vi "Path Variant to Path Array.vi"(8 "error in":errorcluster, 10 "Paths":variant) -> (0 "error out":errorcluster, 2 "Paths":string[](array[string]))   [LabVIEW 2019, in "LV-Data.PGSQL.lvclass"]
uses:
  LV-Data.PGSQL.lvclass
  Typedefs/Errors--enum.ctl
  <vilib>/Utility/Data Type/NI_Data Type.lvlib
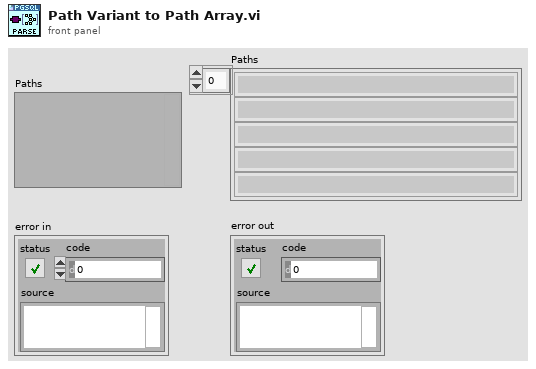
[diagram p1: front panel]
types:
  T1 = typedef "NI_Data Type.lvlib/Data Type.ctl" = enum8{"Invalid Type", "Void", "I8", "I16", "I32", "I64", "U8", "U16", "U32", "U64", "Single Float", "Double Float", "Extended Float", "Single Complex", "Double Complex", "Extended Complex", "Enum U8", "Enum U16", "Enum U32", "Enum U64", "Single Float With Unit", "Double Float With Unit", "Extended Float With Unit", "Single Complex with Unit", "Double Complex with Unit", "Extended Complex with Unit", "Boolean", "String", "Path", "Picture", "Tag", "Array", "Cluster", "Variant", "LV Variant", "Waveform", "Timestamp", "Digital Waveform", "Digital Data", "ExpressData", "Refnum", "External Data", "VI", "Poly VI", "LabVIEW Class Instance", "Fixed Point", "Set Collection", "Map Collection"}
  T2 = typedef "LV-Data.PGSQL.lvclass/Errors--enum.ctl" = enum16{"0: None", "5005: Path Type Not Supported", "5006: Number of Variables", "5007: Number of data points", "5008: Cannot write two data points", "5030: Start and End Times Identical", "5031: Input is not wholly", "5032: Undefined Timestamps", "5033: Bad path or paths", "5040: Invalid Instrument Name", "5050: Column can only hold string", "5051: Column can only hold bool", "5052: Column can only hold double", "5053: Column can only hold int"}
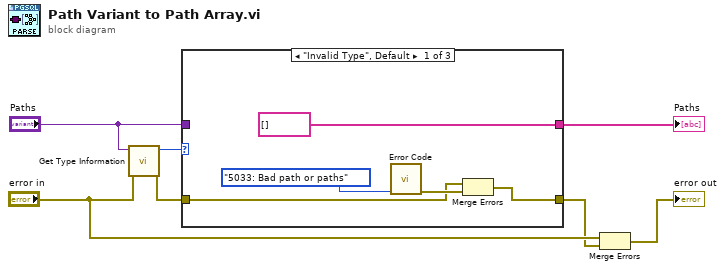
[diagram p0: block diagram]
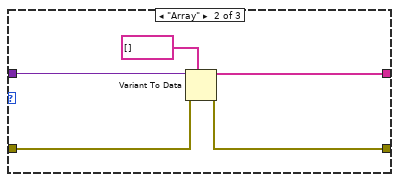
[diagram p2: hidden frame]
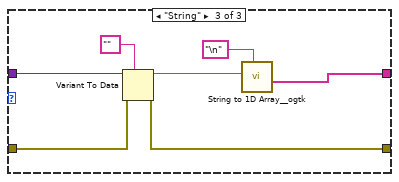
[diagram p3: hidden frame]
diagram:
  n1 = call <vilib>:"Get Type Information.vi"("error in (no error)"="error in", "variant"="Paths") -> ("error out"=w4:errorcluster, "type"=w7:T1)  [unwired: 5 in, 3 out]
  n2 = case shown="\"Invalid Type\", Default" w7 {
    tunnel: "Paths" -> [_ w17 w23]
    tunnel: [string[] [] w15 w21] -> w5
    tunnel: w4 -> [w8 w14 w19]
    tunnel: [w11 w13 w18] -> w2
    frame "Invalid Type", Default {
      n3 = call "Error Code.vi"("Error code"=Errors--enum."5033: Bad path or paths") -> ("error out"=w10:errorcluster)  [unwired: 10 in]
      n4 = Merge Errors(w8, w10) -> (w11:errorcluster)
    }
    frame "Array" {
      n5 = Variant To Data(error in=w14, type=string[] [], Variant=w17) -> (data=w15:string[], error out=w13:errorcluster)
    }
    frame "String" {
      n6 = Variant To Data(error in=w19, type="", Variant=w23) -> (data=w22:string, error out=w18:errorcluster)
      n7 = call <userlib>:"String to 1D Array__ogtk.vi"("delimiter (Tab)"="\n", "string"=w22) -> ("Array of Strings"=w21:string[])  [unwired: 9 in]
    }
  }
  "Paths" <- w5
  n8 = Merge Errors("error in", w2) -> (→"error out":errorcluster)
